vi "NormalToHexString.vi"(7 "Normal Display String":string="01") -> (8 "Hex Display String":string)   [LabVIEW 2015]
doc: "This VI translate the normal display string to hex display string. The two type string display the same."
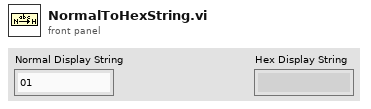
[diagram p1: front panel]
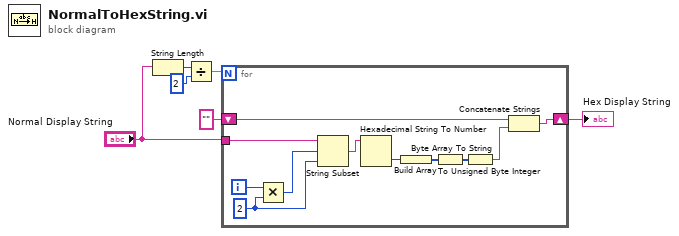
[diagram p0: block diagram]
diagram:
  n1 = String Length(string="Normal Display String") -> (length=w4:i32)
  n2 = Divide(x=w4, y=2 ("length")) -> (x/y=w2:dbl)
  n3 = for {
    N: w2 -> [_]
    tunnel: "Normal Display String" -> [w16]
    shift-right: [w12] -> w1
    shift-left: "" ("String") -> [w13]
    i -> [w11]
    w7 = 2 ("length (rest)")
    n4 = Multiply(x=w11, y=w7) -> (x*y=w10:i32)
    n5 = String Subset(string=w16, offset (0)=w10, length (rest)=w7) -> (substring=w15:string)
    n6 = Hexadecimal String To Number(string=w15) -> (number=w17:u32)  [unwired: 2 in, 1 out]
    n7 = Build Array(w17) -> (w9:u32[])
    n8 = To Unsigned Byte Integer(number=w9) -> (unsigned 8bit integer=w8:u8[])
    n9 = Byte Array To String(unsigned byte array=w8) -> (string=w14:string)
    n10 = Concatenate Strings(w13, w14) -> (w12:string)
  }
  "Hex Display String" <- w1
